vi "reorder cluster.vi"() -> ()   [LabVIEW 2021]
panel:
  in  "cluster":cluster{"a":dbl, "b":dbl, "c":dbl}={"a"=1.0, "b"=2.0, "c"=3.0}
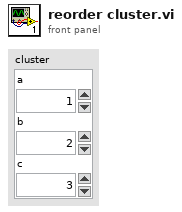
[diagram p1: front panel]
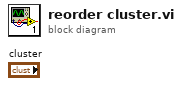
[diagram p0: block diagram]
diagram:
